vi "Check Named Dependency.vi"(8 "error in (no error)":errorcluster, 9 "Args in":string[](array[string]), 11 "AddAction in":refnum<class "AddAction.lvclass">) -> (0 "error out":errorcluster, 1 "Remaining Args":string[](array[string]), 3 "AddAction out":refnum<class "AddAction.lvclass">)   [LabVIEW 2020, in "GPackTools.lvlib" / "AddAction.lvclass"]
uses:
  AddAction.lvclass
  AddAction.lvclass/AddAction.ctl
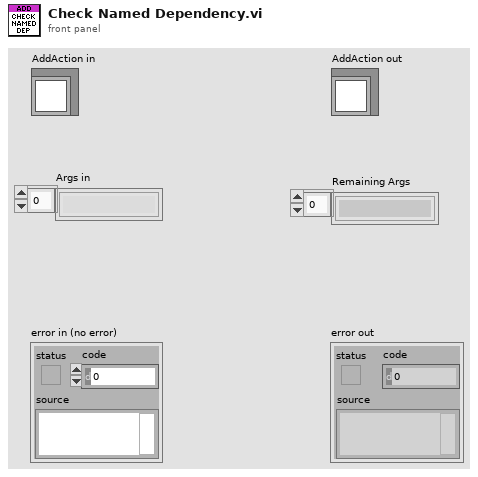
[diagram p1: front panel]
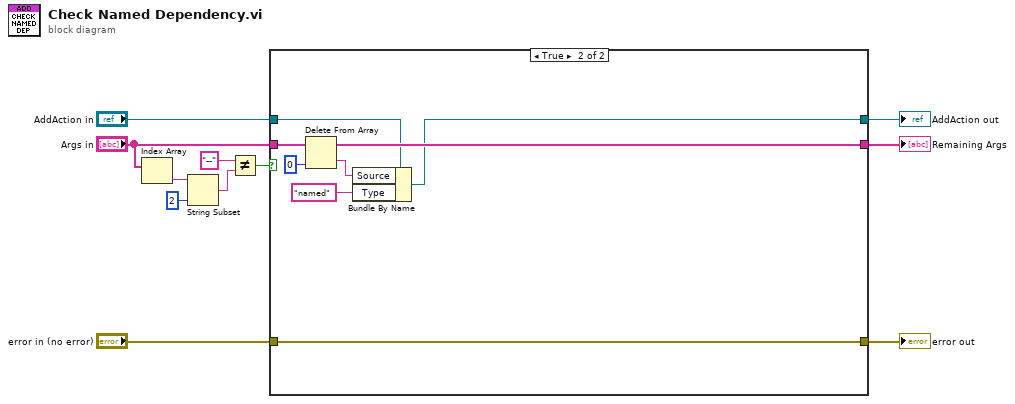
[diagram p0: block diagram]
diagram:
  n1 = Index Array(array="Args in") -> (element=w11:string)  [unwired: 1 in]
  n2 = String Subset(string=w11, length (rest)=2 ("length (rest)")) -> (substring=w9:string)  [unwired: 1 in]
  n3 = Not Equal?(x="--", y=w9) -> (x != y?=w7:bool)
  n4 = case shown="True" w7 {
    tunnel: "AddAction in" -> [w13 w18]
    tunnel: "Args in" -> [w14 w22]
    tunnel: [w14 w20] -> w4
    tunnel: [w13 w15] -> w3
    tunnel: [w12 w19] -> w2
    tunnel: "error in (no error)" -> [w12 w19]
    frame False {
      # "Not a named repo initial argument, pass on as-is for the rest of argument parsing."
    }
    frame True {
      n5 = Delete From Array(array=w22, index=0) -> (deleted portion=w17:string, array with subset deleted=w20:string[])  [unwired: 1 in]
      n6 = Bundle By Name(cluster=w18, "Source"=w17, "Type"="named") -> (w15:refnum<class "AddAction.lvclass">)
    }
  }
  "error out" <- w2
  "AddAction out" <- w3
  "Remaining Args" <- w4
